vi "uart data_akcelerometr_copy_onlyplots.vi"() -> ()   [LabVIEW 2015]
uses:
  data_typedef.ctl
  <vilib>/Instr/_visa.llb/VISA Configure Serial Port (Instr).vi
panel:
  out "Array 2":dbl[](array[numeric])
  out "Accelero Chart":T1(graph)
  out "Temperature Chart":dbl[](graph)
  in  "stop":bool
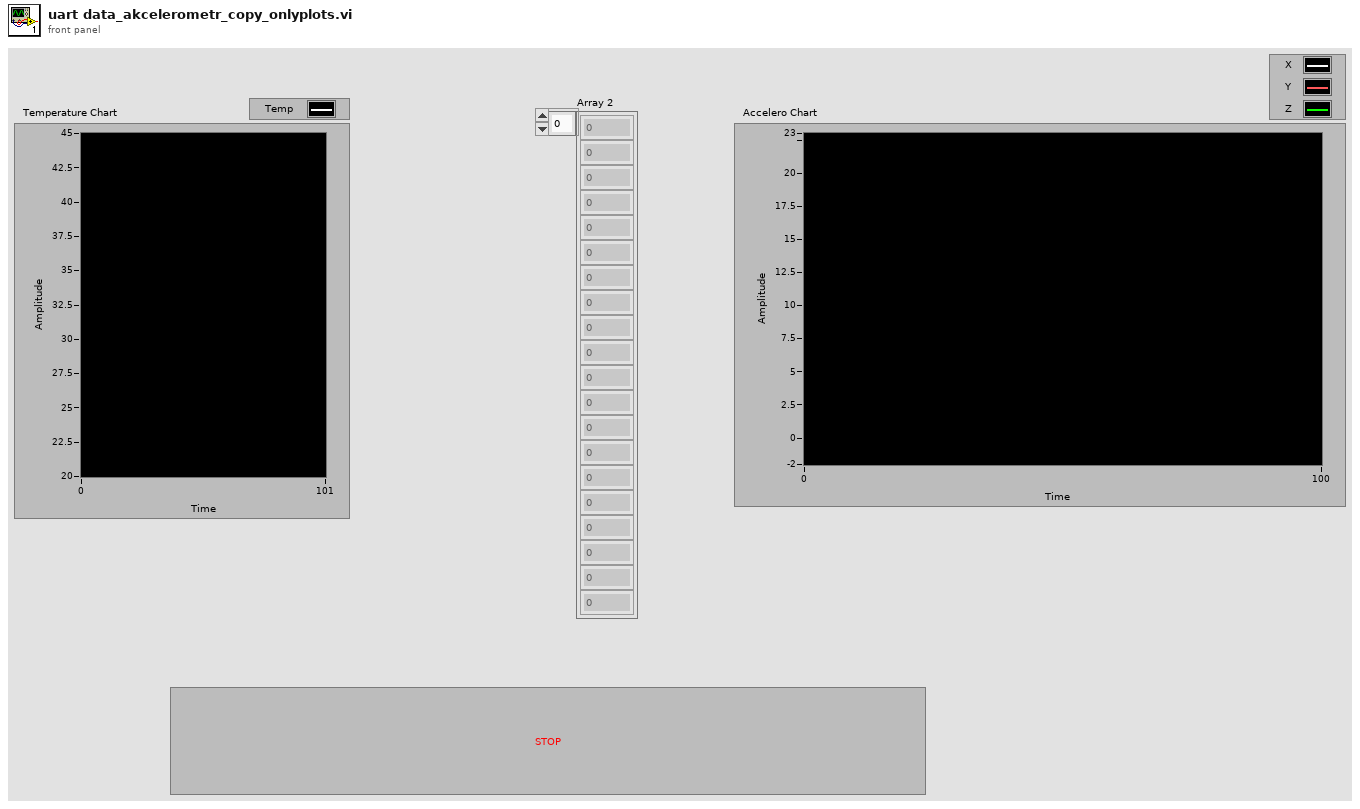
[diagram p1: front panel]
types:
  T1 = cluster{"X element out":dbl, "X element out":dbl, "Z element out":dbl}
  T2 = cluster{"Z element out":dbl, "X element out":dbl, "X element out 2":dbl}[]
  T3 = typedef "data_typedef.ctl" = cluster{"Accelero Array":dbl[], "Z out":dbl[], "Y out":dbl[], "X out":dbl[], "Numeric":i32}
  T4 = typedef "enum_typedef.ctl" = enum16{"Temperature", "X axis", "Y axis", "Z axis"}
  T5 = cluster{"X element out":dbl, "Y element out":dbl, "Z element out":dbl}
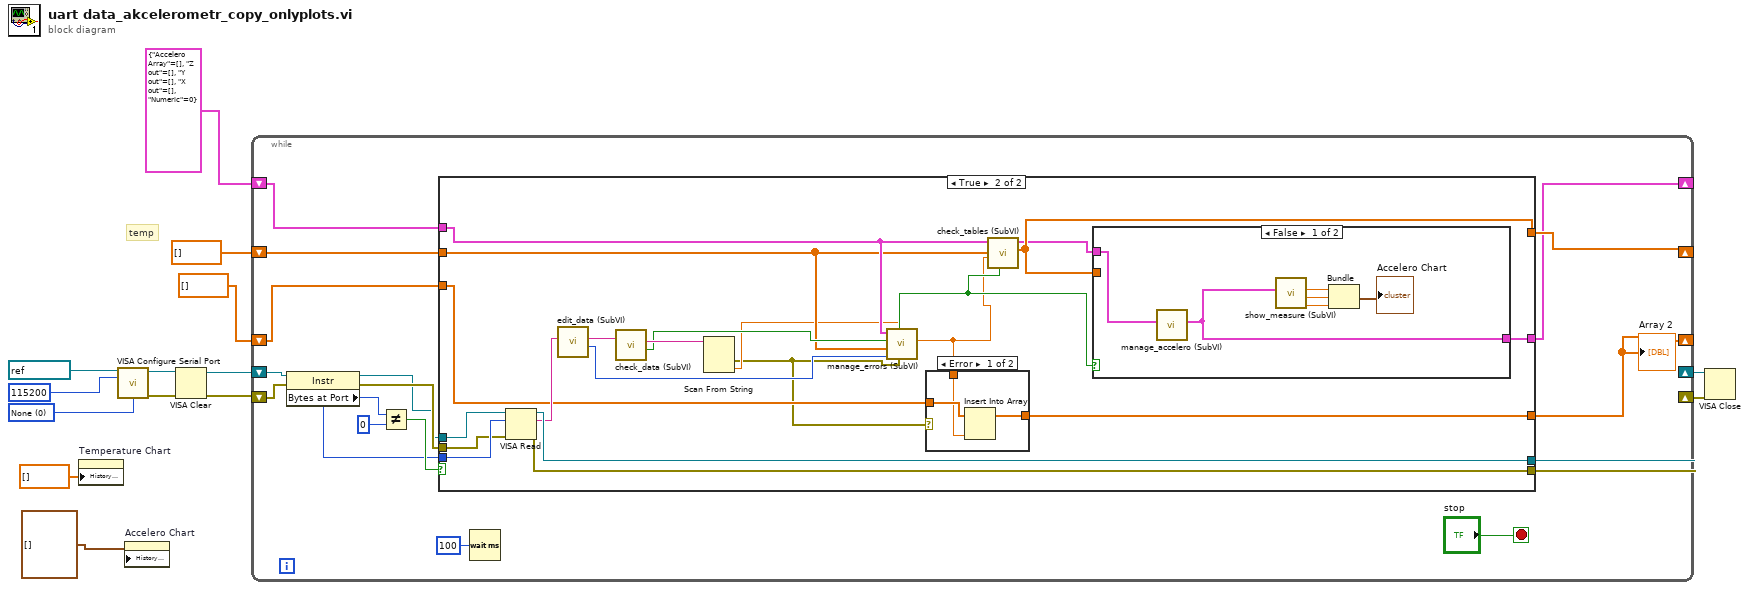
[diagram p0: block diagram]
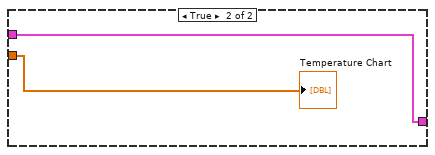
[diagram p4: hidden frame]
diagram:
  w10 = u16 0 items=["None", "XON/XOFF", "RTS/CTS", "XON/XOFF & RTS/CTS", "DTR/DSR", "XON/XOFF & DTR/DSR"] ("flow control (0:none)")
  # "temp"
  n1 = property on="Temperature Chart" class="WFChart (strict)"("History Data"=dbl[] []) -> ()  [unwired: 2 in, 2 out]
  n2 = call-poly "VISA Configure Serial Port"("VISA resource name"=refnum<visa-resource-name> "COM5", "baud rate (9600)"=u32 115200, "flow control (0:none)"=w10) -> ("VISA resource name out"=w6:refnum<visa-resource-name>, "error out"=w5:errorcluster)  [unwired: 11 in]
  n3 = property on="Accelero Chart" class="WFChart (strict)"("History Data"=T2 []) -> ()  [unwired: 2 in, 2 out]
  n4 = VISA Clear(VISA resource name=w6, error in (no error)=w5) -> (VISA resource name out=w7:refnum<visa-resource-name>, error out=w8:errorcluster)
  n5 = while {
    shift-right: [w30] -> w12
    shift-left: w7 -> [w29]
    shift-right: [w26] -> w11
    shift-left: w8 -> [w27]
    shift-right: [w19] -> _
    shift-left: dbl[] [] -> [w22]
    shift-right: [w17] -> _
    shift-left: T3 {"Accelero Array"=[], "Z out"=[], "Y out"=[], "X out"=[], "Numeric"=0} ("Tabs") -> [w18]
    shift-right: [w15] -> _
    shift-left: dbl[] [] -> [w16]
    stop <- "stop" stop-if-true
    # "main loop"
    n6 = property class="Instr"(reference=w29, error in=w27) -> (reference out=w25:refnum<visa-resource-name>, error out=w28:errorcluster, "Bytes at Port"=w21:u32)
    n7 = Not Equal?(x=w21, y=u32 0) -> (x != y?=w23:bool)
    n8 = case shown="True" w23 {
      tunnel: [w36 w57] -> w30
      tunnel: w21 -> [_ w56]
      tunnel: w28 -> [w35 w55]
      tunnel: [w35 w54] -> w26
      tunnel: w25 -> [w36 w53]
      tunnel: w22 -> [w34 w41]
      tunnel: [w34 w50] -> w19
      tunnel: w18 -> [w33 w42]
      tunnel: [w33 w49] -> w17
      tunnel: w16 -> [w32 w46]
      tunnel: [w32 w45] -> w15
      frame False {
      }
      frame True {
        # "true"
        n9 = VISA Read(VISA resource name=w53, byte count=w56, error in (no error)=w55) -> (VISA resource name out=w57:refnum<visa-resource-name>, read buffer=w52:string, error out=w54:errorcluster)  [unwired: 1 out]
        n10 = call "edit_data (SubVI).vi"("data in"=w52) -> ("Enum"=w44:T4, "data out"=w51:string)  [unwired: 9 in]
        n11 = call "check_data (SubVI).vi"("read buffer"=w51) -> ("buffer out"=w47:string, "bool out"=w43:bool)  [unwired: 8 in]
        n12 = Scan From String(input string=w47) -> (error out=w38:errorcluster, output 1=w39:dbl)  [unwired: 4 in, 2 out]
        n13 = call "manage_errors (SubVI).vi"("error in (no error)"=w38, "Value in"=w39, "Enum"=w44, "Temperature Array"=w41, "Boolean"=w43, "Data in"=w42) -> ("Boolean out"=w40:bool, "Out value"=w37:dbl)  [unwired: 4 in]
        n14 = case shown="Error" w38 {
          tunnel: w46 -> [w60 w61]
          tunnel: [w59 w61] -> w45
          tunnel: w37 -> [w58 _]
          frame Error {
            n15 = Insert Into Array(array=w60, new element=w58) -> (w59:dbl[])  [unwired: 1 in]
          }
          frame No Error {
          }
        }
        n16 = call "check_tables (SubVI).vi"("bool in"=w40, "numeric buffer in"=w37, "temperature array in"=w41, "Data in"=w42) -> ("temperature array out"=w50:dbl[], "Data out"=w48:T3)  [unwired: 6 in]
        n17 = case shown="False" w40 {
          tunnel: w50 -> [_ w69]
          tunnel: w48 -> [w63 w68]
          tunnel: [w62 w68] -> w49
          frame False {
            n18 = call "manage_accelero (SubVI).vi"("Data in"=w63) -> ("Data out"=w62:T3)  [unwired: 9 in]
            n19 = call "show_measure (SubVI).vi"("Data in"=w62) -> ("Z element out"=w66:dbl, "Y element out"=w64:dbl, "X element out"=w67:dbl)  [unwired: 8 in]
            n20 = Bundle("X element out"=w67, "Y element out"=w64, "Z element out"=w66) -> (→"Accelero Chart":T5)  [unwired: 1 in]
          }
          frame True {
            "Temperature Chart" <- w69
          }
        }
      }
    }
    "Array 2" <- w15
    n21 = Wait (ms)(milliseconds to wait=u32 100) -> ()  [unwired: 1 out]
  }
  n22 = VISA Close(VISA resource name=w12, error in (no error)=w11) -> ()  [unwired: 1 out]
